vi "Create  (TagCircle49h12).vi"(8 "error in (no error)":errorcluster, 11 "Detector Settings":T1={"Refine Edges (Default: True)"=TRUE, "Threads (Default: 1)"=1, "Decimate (Default: 1)"=1.0, "Blur (Default: 0)"=0.0, "Bits (Default: 2)"=2} {"Threads (Default: 1)" min=1}) -> (0 "error out":errorcluster, 3 "New Apriltag Detector":refnum<class "AprilTag Detector.lvclass">)   [LabVIEW 2020, in "g_ar_toolkit.feature_detection.lvlib" / "AprilTag Detector.lvclass"]
uses:
  AprilTag Detector.lvclass
  Detector Settings.ctl
  AprilTag Families.ctl
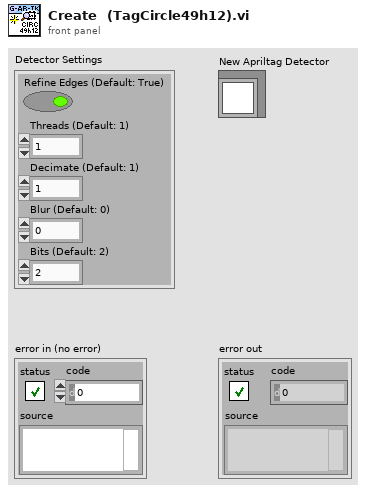
[diagram p1: front panel]
types:
  T1 = typedef "g_ar_toolkit.feature_detection.lvlib/AprilTag Detector.lvclass/Detector Settings.ctl" = cluster{"Refine Edges (Default: True)":bool, "Threads (Default: 1)":u8, "Decimate (Default: 1)":sgl, "Blur (Default: 0)":sgl, "Bits (Default: 2)":u8}
  T2 = typedef "g_ar_toolkit.feature_detection.lvlib/AprilTag Detector.lvclass/AprilTag Families.ctl" = enum8{"tag16h5", "tag25h9", "tag36h11", "tagCircle21h7", "tagCircle49h12", "tagCustom48h12", "tagStandard41h12", "tagStandard52h13"}
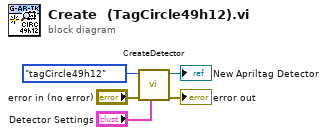
[diagram p0: block diagram]
diagram:
  n1 = call "CreateDetector.vi"("Detector Settings"="Detector Settings", "error in (no error)"="error in (no error)", "Family"=AprilTag_Families."tagCircle49h12") -> ("error out"=→"error out":errorcluster, "New Apriltag Detector"=→"New Apriltag Detector":refnum<class "AprilTag Detector.lvclass">)  [unwired: 7 in]
